vi "Retrieve_latest_PAQ_data.vi"(8 "error in (no error)":errorcluster, 10 "FetchLatestDefinition":T2, 11 "DBAL-SQLite in":refnum<class "DBAL-SQLite.lvclass">) -> (0 "error out":errorcluster, 2 "BinHistData":T1, 3 "DBAL-SQLite out":refnum<class "DBAL-SQLite.lvclass">)   [LabVIEW 2020, in "Sgraph_lib_V1.lvlib" / "DBAL-SQLite.lvclass"]
uses:
  DBAL-SQLite.lvclass
  controls/DBAL_FetchLatestFrom.ctl
  controls/BIN/BINdata.ctl
  DBAL.lvclass
  DBAL-BIN.lvclass
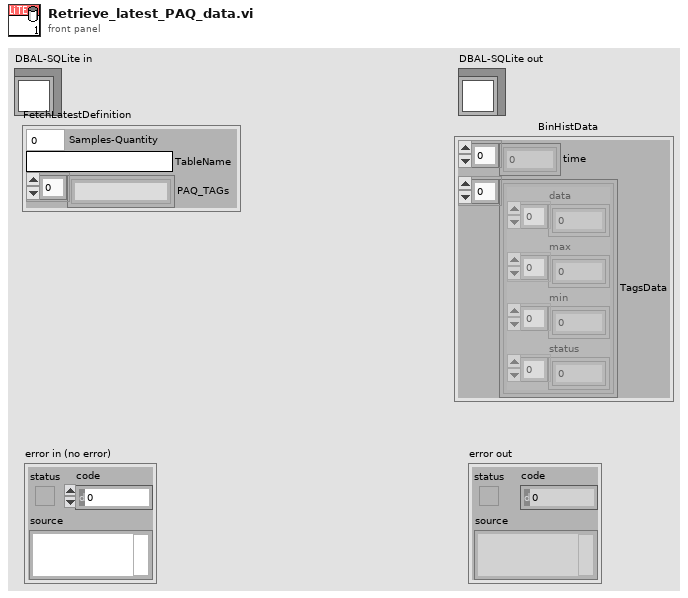
[diagram p1: front panel]
types:
  T1 = typedef "Sgraph_lib_V1.lvlib/DBAL-BIN.lvclass/BINdata.ctl" = cluster{"time":dbl[], "TagsData":cluster{"data":dbl[], "max":dbl[], "min":dbl[], "status":u32[]}[]}
  T2 = typedef "Sgraph_lib_V1.lvlib/DBAL.lvclass/DBAL_FetchLatestFrom.ctl" = cluster{"Samples-Quantity":i32, "TableName":string, "PAQ_TAGs":string[]}
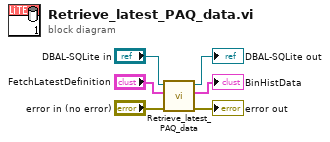
[diagram p0: block diagram]
diagram:
  n1 = call-parent "Retrieve_latest_PAQ_data.vi"("error in (no error)"="error in (no error)", "FetchLatestDefinition"="FetchLatestDefinition", "DBAL in"="DBAL-SQLite in") -> ("error out"=→"error out":errorcluster, "BinHistData"=→"BinHistData":T1, "DBAL out"=→"DBAL-SQLite out":refnum<class "DBAL-SQLite.lvclass">)  [unwired: 6 in]
